vi "בדיקת צריכת זרם של סליל הפיקוד Mod.vi"(7 "resultUserPrompt":bool, 8 "error":errorcluster, 9 "זרם מקסימלי":dbl=0.105 format="%#_13g", 10 "שם הממסר":string="0410-24534 15A ממסר", 11 "Path for Log":path) -> (0 "error out":errorcluster, 2 "צריכת זרם בסליל בטווח כן/לא":bool, 3 "צריכת זרם בסליל":dbl format="%.4f")   [LabVIEW 2014]
uses:
  <vilib>/DAQmx/create/channels.llb/DAQmx Create Channel (DO-Digital Output).vi
  <vilib>/DAQmx/write.llb/DAQmx Write (Digital Bool 1Line 1Point).vi
panel:
  # "Right-Click to\nexplain error"
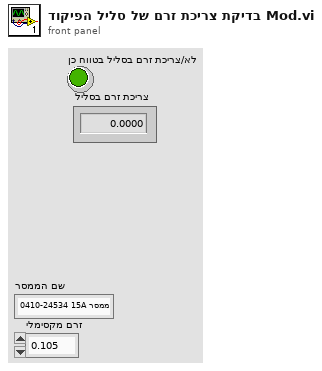
[diagram p1: front panel]
types:
  T1 = enum32{"Invalid", "Standard", "Closed", "Hidden", "Minimized", "Maximized"}
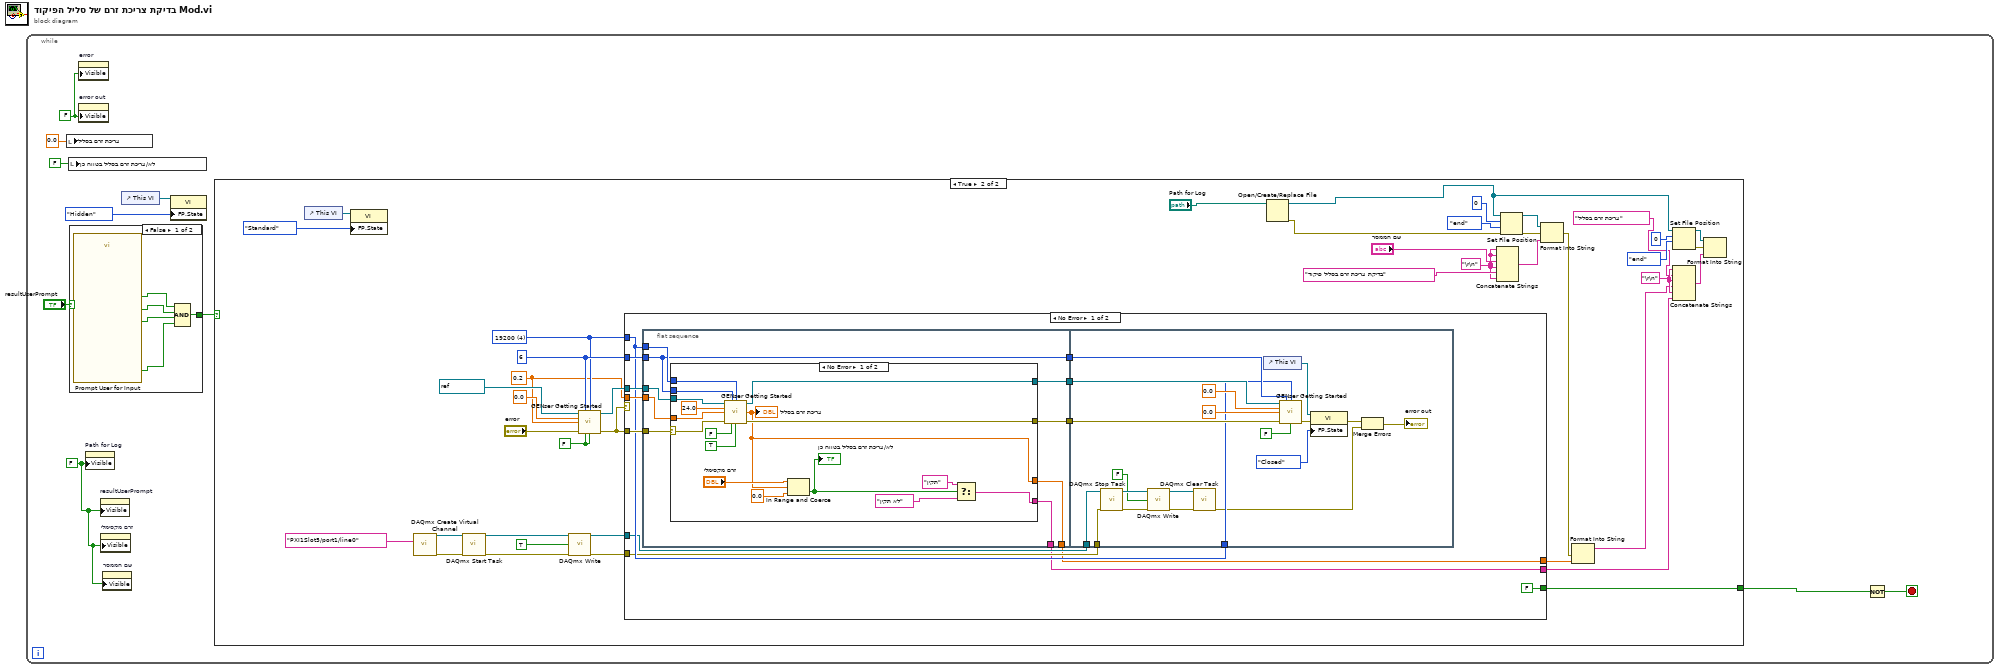
[diagram p0: block diagram]
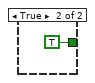
[diagram p2: hidden frame]
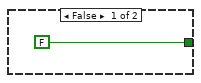
[diagram p3: hidden frame]
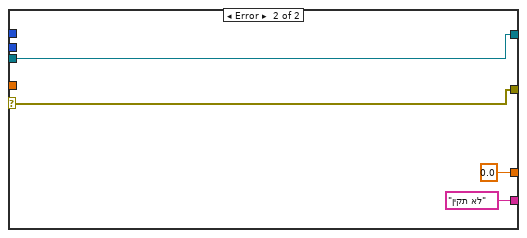
[diagram p4: hidden frame]
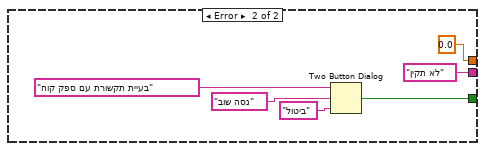
[diagram p5: hidden frame]
diagram:
  n1 = while {
    stop <- w10 stop-if-true
    w1 = FALSE ("Visible")
    w5 = FALSE ("Visible")
    n2 = local write "צריכת זרם בסליל"(0.0 ("Output Current")) -> ()
    n3 = local write "צריכת זרם בסליל בטווח כן/לא"(FALSE ("In Range?")) -> ()
    n4 = case shown="False" "resultUserPrompt" {
      tunnel: [w15 TRUE] -> w8
      frame False {
        n5 = call "Prompt User for Input"() -> ("הדקי הרב מודד"=w11:bool, "מגע שלילי"=w12:bool, "מגע חיובי"=w13:bool, "OK"=w14:bool)  [unwired: 15 in, 1 out]
        n6 = Compound Arithmetic op=AND(w14, w13, w12, w11) -> (w15:bool)
      }
      frame True {
      }
    }
    n7 = property on="error" class="Clust (strict)"("Visible"=w5) -> ()  [unwired: 2 in, 2 out]
    n8 = property on="error out" class="Clust (strict)"("Visible"=w5) -> ()  [unwired: 2 in, 2 out]
    n9 = property on="Path for Log" class="Path"("Visible"=w1) -> ()  [unwired: 2 in, 2 out]
    n10 = property on="resultUserPrompt" class="Bool (strict)"("Visible"=w1) -> ()  [unwired: 2 in, 2 out]
    n11 = property on="זרם מקסימלי" class="DigNum (strict)"("Visible"=w1) -> ()  [unwired: 2 in, 2 out]
    n12 = property on="שם הממסר" class="Str"("Visible"=w1) -> ()  [unwired: 2 in, 2 out]
    n13 = control-ref of="This VI"() -> (w4:refnum<vi>)
    n14 = property class="VI"(reference=w4, "FP.State"=T1."Hidden" ("Front Panel Window:State")) -> ()  [unwired: 1 in, 2 out]
    n15 = case shown="True" w8 {
      tunnel: [FALSE ("T button?") w51] -> w9
      frame False {
      }
      frame True {
        w24 = "\r\n"
        w33 = "\r\n"
        w50 = FALSE ("Output On (T)")
        w55 = u16 4 items=["1200", "2400", "4800", "9600", "19200"] ("BAUD")
        w56 = i16 6 ("GEN Addr")
        w52 = 0.2 ("Current Limit")
        n16 = control-ref of="This VI"() -> (w49:refnum<vi>)
        n17 = property class="VI"(reference=w49, "FP.State"=T1."Standard" ("Front Panel Window:State")) -> ()  [unwired: 1 in, 2 out]
        n18 = call-poly <vilib>:"DAQmx Create Virtual Channel.vi"("lines"=tag "PXI1Slot5/port1/line0") -> ("task out"=w46:refnum<k21>, "error out"=w47:errorcluster)  [unwired: 13 in]
        n19 = call <vilib>:"DAQmx Start Task.vi"("task/channels in"=w46, "error in"=w47) -> ("task out"=w44:refnum<k21>, "error out"=w43:errorcluster)  [unwired: 12 in]
        n20 = call-poly <vilib>:"DAQmx Write.vi"("task/channels in"=w44, "data"=TRUE, "error in"=w43) -> ("task out"=w41:refnum<k21>, "error out"=w40:errorcluster)  [unwired: 10 in, 1 out]
        n21 = call "GENser Getting Started.vi"("VISA"=refnum<visa-resource-name> "COM6", "GEN Addr"=w56, "BAUD"=w55, "Voltage Limit"=0.0, "Current Limit"=w52, "error"="error", "Reset (T)"=w50, "Output On (T)"=w50) -> ("VISA out"=w57:refnum<visa-resource-name>, "error out"=w58:errorcluster)  [unwired: 4 in, 2 out]
        n22 = case shown="No Error" w58 {
          tunnel: w58 -> [w67 _]
          tunnel: w57 -> [w69 _]
          tunnel: w56 -> [w70 _]
          tunnel: w55 -> [w64 _]
          tunnel: w52 -> [w68 _]
          tunnel: [FALSE w125] -> w51
          tunnel: w41 -> [w63 _]
          tunnel: w40 -> [w62 _]
          tunnel: [w61 0.0 ("Output Current")] -> w30
          tunnel: [w60 "לא תקין"] -> w22
          frame No Error {
            n23 = flat-sequence {
              tunnel: [w81] -> w71
              tunnel: w64 -> [w80]
              tunnel: w70 -> [w76]
              tunnel: w69 -> [w79]
              tunnel: w68 -> [w78]
              tunnel: w67 -> [w75]
              tunnel: [w77] -> w66
              tunnel: [w76] -> w65
              tunnel: [w74] -> w61
              tunnel: [w73] -> w60
              tunnel: w71 -> [w119]
              tunnel: w66 -> [w118]
              tunnel: w65 -> [w117]
              tunnel: w64 -> [w116]
              tunnel: w63 -> [w104]
              tunnel: w62 -> [w103]
              frame #0 {
                n24 = case shown="No Error" w75 {
                  selector: w75 -> [w87 w101]
                  tunnel: [w93 w101] -> w81
                  tunnel: w80 -> [w92 _]
                  tunnel: w76 -> [w91 _]
                  tunnel: w79 -> [w90 w102]
                  tunnel: w78 -> [w89 _]
                  tunnel: [w88 w102] -> w77
                  tunnel: [w86 0.0 ("Output Current")] -> w74
                  tunnel: [w82 "לא תקין"] -> w73
                  frame No Error {
                    n25 = call "GENser Getting Started.vi"("VISA"=w90, "GEN Addr"=w91, "BAUD"=w92, "Voltage Limit"=24.0, "Current Limit"=w89, "error"=w87, "Reset (T)"=FALSE, "Output On (T)"=TRUE) -> ("VISA out"=w88:refnum<visa-resource-name>, "Output Current"=w86:dbl, "error out"=w93:errorcluster)  [unwired: 4 in, 1 out]
                    "צריכת זרם בסליל" <- w86
                    n26 = In Range and Coerce(upper limit="זרם מקסימלי", x=w86, lower limit=0.0) -> (In Range?=w83:bool)  [unwired: 1 out]
                    "צריכת זרם בסליל בטווח כן/לא" <- w83
                    n27 = Select(t="תקין", s=w83, f="לא תקין") -> (s? t:f=w82:string)
                  }
                  frame Error {
                  }
                }
              }
              frame #1 {
                n28 = call <vilib>:"DAQmx Stop Task.vi"("task/channels in"=w104, "error in"=w103) -> ("task out"=w112:refnum<k21>, "error out"=w111:errorcluster)  [unwired: 12 in]
                n29 = call-poly <vilib>:"DAQmx Write.vi"("task/channels in"=w112, "data"=FALSE, "error in"=w111) -> ("task out"=w110:refnum<k21>, "error out"=w109:errorcluster)  [unwired: 10 in, 1 out]
                n30 = call <vilib>:"DAQmx Clear Task.vi"("task in"=w110, "error in"=w109) -> ("error out"=w106:errorcluster)  [unwired: 13 in]
                n31 = control-ref of="This VI"() -> (w115:refnum<vi>)
                n32 = call "GENser Getting Started.vi"("VISA"=w118, "GEN Addr"=w117, "BAUD"=w116, "Voltage Limit"=0.0, "Current Limit"=0.0, "error"=w119, "Output On (T)"=FALSE) -> ("error out"=w113:errorcluster)  [unwired: 5 in, 3 out]
                n33 = property class="VI"(reference=w115, error in=w113, "FP.State"=T1."Closed" ("Front Panel Window:State")) -> (error out=w107:errorcluster)  [unwired: 1 out]
                n34 = Merge Errors(w107, w106) -> (→"error out":errorcluster)
              }
            }
          }
          frame Error {
            n35 = Two Button Dialog(message="בעיית תקשורת עם ספק קוח", 1:"ביטול" ("F button name (\"Cancel\")"), 2:"נסה שוב" ("T button name (\"OK\")")) -> (T button?=w125:bool)
          }
        }
        n36 = Open/Create/Replace File(file path (use dialog)="Path for Log") -> (refnum out=w18:refnum<file>, error out=w19:errorcluster)  [unwired: 5 in, 1 out]
        n37 = Concatenate Strings(w33, w33, "שם הממסר", w33, "בדיקת צריכת זרם בסליל פיקוד", w33) -> (w37:string)
        n38 = Set File Position(offset (in bytes) (0)=i64 0, refnum=w18, from (0:start)=enum16{"start", "end", "current"}."end", error in=w19) -> (refnum out=w34:refnum<file>, error out=w32:errorcluster)
        n39 = Format Into String(initial string=w34, error in=w32, w37) -> (error out=w31:errorcluster)  [unwired: 1 in, 1 out]
        n40 = Format Into String(error in=w31, w30) -> (resulting string=w21:string)  [unwired: 2 in, 1 out]
        n41 = Set File Position(offset (in bytes) (0)=i64 0, refnum=w18, from (0:start)=enum16{"start", "end", "current"}."end") -> (refnum out=w27:refnum<file>, error out=w28:errorcluster)  [unwired: 1 in]
        n42 = Concatenate Strings(w24, "צריכת זרם בסליל", w24, w21, w24, w22) -> (w29:string)
        n43 = Format Into String(initial string=w27, error in=w28, w29) -> ()  [unwired: 1 in, 2 out]
      }
    }
    n44 = Not(x=w9) -> (.not. x?=w10:bool)
  }
